vi "Cycle.vi"(8 "error in (no error)":errorcluster, 11 "TwoAFCeye In":refnum<class "TwoAFCeye.lvclass">) -> (0 "error out":errorcluster, 3 "TwoAFCeye Out":refnum<class "TwoAFCeye.lvclass">)   [LabVIEW 2010, in "TwoAFCeye.lvclass"]
uses:
  TwoAFCeye.lvclass
  MatlabExperiment/MatlabExperiment.lvclass
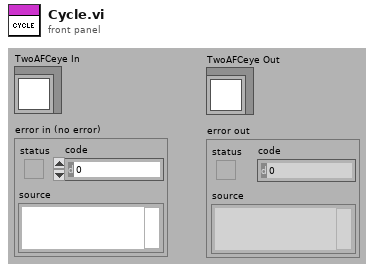
[diagram p1: front panel]
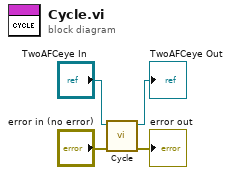
[diagram p0: block diagram]
diagram:
  n1 = call-parent "Cycle.vi"("error in (no error)"="error in (no error)", "MatlabExperiment In"="TwoAFCeye In") -> ("error out"=→"error out":errorcluster, "MatlabExperiment Out"=→"TwoAFCeye Out":refnum<class "TwoAFCeye.lvclass">)  [unwired: 8 in]
